vi "uA_daq_Capture_Current_waveform_to_new_chart.vi"(9 "Sample rate":dbl, 10 "CrsrList":T1, 11 "Waveform_main":waveform(sgl)) -> (1 "Numeric":dbl, 2 "Waveform":waveform(sgl), 3 "Numeric 2":sgl)   [LabVIEW 2015]
uses:
  <vilib>/Utility/miscctls.llb/LVCursorListTypeDef.ctl
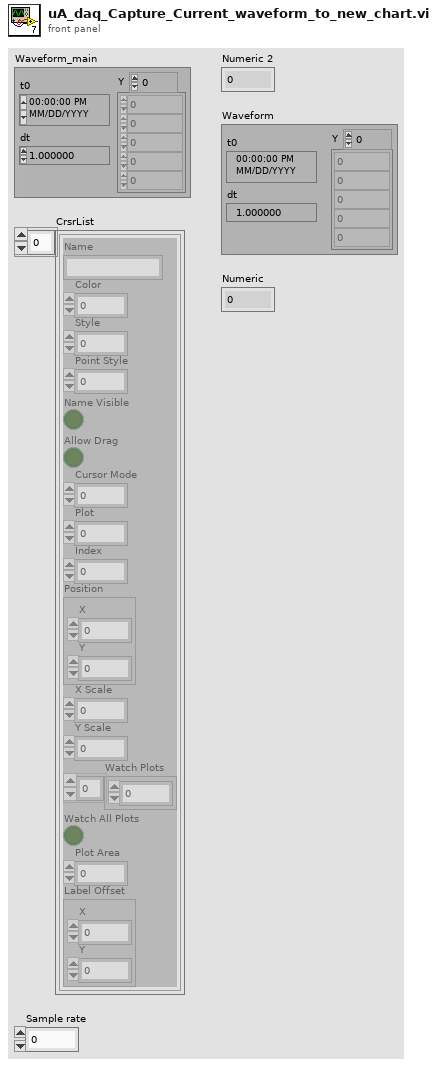
[diagram p1: front panel]
types:
  T1 = typedef "LVCursorListTypeDef.ctl" = cluster{"Name":string, "Color":u32, "Style":u8, "Point Style":u8, "Name Visible":bool, "Allow Drag":bool, "Cursor Mode":u32, "Plot":i32, "Index":i32, "Position":cluster{"X":dbl, "Y":dbl}, "X Scale":u32, "Y Scale":u32, "Watch Plots":i32[], "Watch All Plots":bool, "Plot Area":i32, "Label Offset":cluster{"X":dbl, "Y":dbl}}[]
  T2 = cluster{"Name":string, "Color":u32, "Style":u8, "Point Style":u8, "Name Visible":bool, "Allow Drag":bool, "Cursor Mode":u32, "Plot":i32, "Index":i32, "Position":cluster{"X":dbl, "Y":dbl}, "X Scale":u32, "Y Scale":u32, "Watch Plots":i32[], "Watch All Plots":bool, "Plot Area":i32, "Label Offset":cluster{"X":dbl, "Y":dbl}}
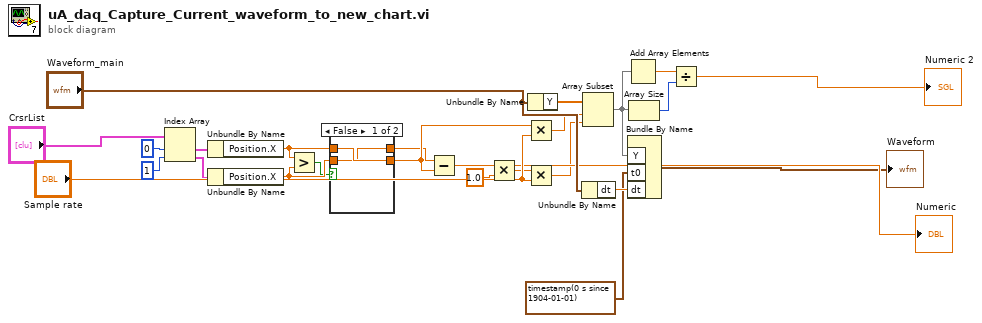
[diagram p0: block diagram]
diagram:
  n1 = Index Array(array="CrsrList", index #1=0 ("index"), index #2=1 ("index")) -> (element #1=w11:T2, element #2=w16:T2)
  n2 = Unbundle By Name(w11) -> ("Position.X"=w19:dbl)
  n3 = Unbundle By Name(w16) -> ("Position.X"=w18:dbl)
  n4 = Greater?(x=w19, y=w18) -> (0:w17:bool)
  n5 = case shown="False" w17 {
    tunnel: w19 -> [w27 w29]
    tunnel: w18 -> [w26 w28]
    tunnel: [w26 w29] -> w20
    tunnel: [w27 w28] -> w21
    frame False {
    }
    frame True {
    }
  }
  n6 = Subtract(x=w20, y=w21) -> (x-y=w22:dbl)
  "Numeric" <- w22
  n7 = Multiply(x=w22, y=1.0) -> (x*y=w10:dbl)
  n8 = Multiply(x=w21, y="Sample rate") -> (x*y=w2:dbl)
  n9 = Multiply(x=w10, y="Sample rate") -> (x*y=w3:dbl)
  n10 = Unbundle By Name("Waveform_main") -> ("Y"=w24:sgl[])
  n11 = Unbundle By Name("Waveform_main") -> ("dt"=w5:dbl)
  n12 = Array Subset(array=w24, index=w2, length=w3) -> (w6:sgl[])
  n13 = Add Array Elements(numeric array=w6) -> (sum=w7:sgl)
  n14 = Bundle By Name("Y"=w6, "t0"=timestamp(0 s since 1904-01-01), "dt"=w5) -> (→"Waveform":waveform(sgl))  [unwired: 1 in]
  n15 = Array Size(array=w6) -> (size(s)=w8:i32)
  n16 = Divide(x=w7, y=w8) -> (x/y=→"Numeric 2":sgl)
